vi "Draw_rectangle.vi"(11 "Coords":cluster{i32, i32}) -> (3 "rect":cluster{i32, i32, i32, i32})   [LabVIEW 2010]
doc: "This VI implements the routine for generating the coords to draw a rectangle of 10x10 pix in the coords specified.\n\nCreated by Davis Montenegro\n06-30-2017"
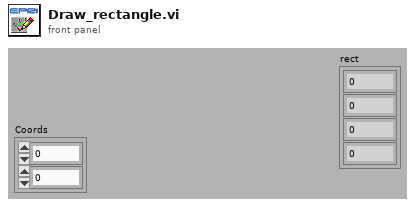
[diagram p1: front panel]
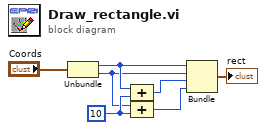
[diagram p0: block diagram]
diagram:
  w6 = 10 ("value")
  n1 = Unbundle("Coords") -> (w5:i32, w4:i32)
  n2 = Compound Arithmetic op=ADD(w5, w6) -> (w3:i32)
  n3 = Compound Arithmetic op=ADD(w4, w6) -> (w2:i32)
  n4 = Bundle(w5, w4, w3, w2) -> (→"rect":cluster{i32, i32, i32, i32})  [unwired: 1 in]
